vi "MyHostCode.vi"() -> ()   [LabVIEW 2017]
doc: "This VI was generated automatically using the FPGA Wizard. You can modify the VI normally."
uses:
  <vilib>/rvi/interface/nirviMethod/nirviMethod.xnode
  <vilib>/rvi/interface/nirviCloseFPGA/nirviCloseFPGA.xnode
  <vilib>/rvi/interface/nirviOpenFPGA/nirviOpenFPGA.xnode
  <vilib>/rvi/interface/nirviReadWriteControl/nirviReadWriteControl.xnode
  <vilib>/rvi/errors/niLvFpgaAdjustHostInterfaceError.vi
  <vilib>/rvi/interface/Simulation/niFpgaSimulationCallBeginRW.vi
  <vilib>/FPGAPlugInAG/Dynamic/niLvFpga_ReadFifo_Dynamic.vi
  <vilib>/rvi/errors/niLvFpgaMergeErrorWithErrorCode.vi
  HostCode.lvlib
  <vilib>/Utility/file.llb/Write To Spreadsheet File (I64).vi
  SerialComm/SerialComm.lvclass
  C:/Program Files (x86)/National Instruments/LabVIEW 2017/examples/Instrument IO/Serial/support/Serial - Settings.ctl
  FPGA Bitfiles/ECGPWMAdaptiveFi_FPGATarget2_ECGAFSPIInput_RcPp5Qijrrw.lvbitx
  FPGACode/ECG AF SPI Input.vi
  <vilib>/FPGAPlugInAG/Dynamic/niLvFpga_Reset_Dynamic.vi
  <vilib>/FPGAPlugInAG/Dynamic/niLvFpga_Run_Dynamic.vi
  <vilib>/FPGAPlugInAG/Dynamic/niLvFpga_Close_Dynamic.vi
  FPGACode/Lead Enum.ctl
  Trigger Params.ctl
  FPGACode/Channel Enum.ctl
panel:
  in  "Offset":cluster{"X":i16, "Y":i16, "Z":i16}
  in  "Beta IBP":fxp<+/-,32,-16>
  out "Pressure Data":T1(array[cluster])
  in  "ECG Gain":u16(ring)=1 items=["1"=1, "2"=2, "3"=3, "4"=4, "6"=0, "8"=5, "12"=6]
  in  "Channel":i32
  in  "Sensis\nECG Scaling":i16=1 min=1 max=100 step=1
  out "RA":i16[](graph)
  out "Trigger":i16[][](graph)
  in  "Trigger":T2={"Channel"=enum."II", "Threshold"=1000, "d/dt"=FALSE, "Invert"=FALSE}
  in  "High Pass":bool
  out "Loop Time":u32
  in  "Reset":bool
  out "Taps":dbl[](graph)
  out "Weights":dbl[](graph)
  out "WeightSum":fxp<+/-,33,19> format="%.20g"
  out "BetaProduct":fxp<+/-,32,-1> format="%.33g"
  in  "Filter Size":i16=100
  out "Invasive Blood Pressure":i16[][](graph)
  in  "Plot Info":T5={"Element"={"Lead"=enum."RA", "Filter"=FALSE}, "Element 2"={"Lead"=enum."RA", "Filter"=TRUE}, "Element 3"={"Lead"=enum."LA", "Filter"=FALSE}, "Element 4"={"Lead"=enum."LA", "Filter"=TRUE}, "Element 5"={"Lead"=enum."LL", "Filter"=FALSE}, "Element 6"={"Lead"=enum."LL", "Filter"=TRUE}, "Element 7"={"Lead"=enum."II", "Filter"=TRUE}, "Element 8"={"Lead"=enum."III", "Filter"=TRUE}}
  in  "file path (dialog if empty)":path
  in  "Record":bool
  out "Gradients":i16[][](graph)
  in  "Filter On":bool=TRUE
  out "ECG":i16[][](graph)
  out "Actual Loop Rate (Ticks)":u32
  in  "Beta":fxp<+/-,32,-16>=1.000088900582341e-11
  out "Late? Latched":bool
  in  "Start 0":bool
  in  "Loop Rate (Hz)":dbl=10000.0
  out "Calculated Rate (Hz)":dbl
  out "error out":errorcluster
  in  "Global Stop":bool
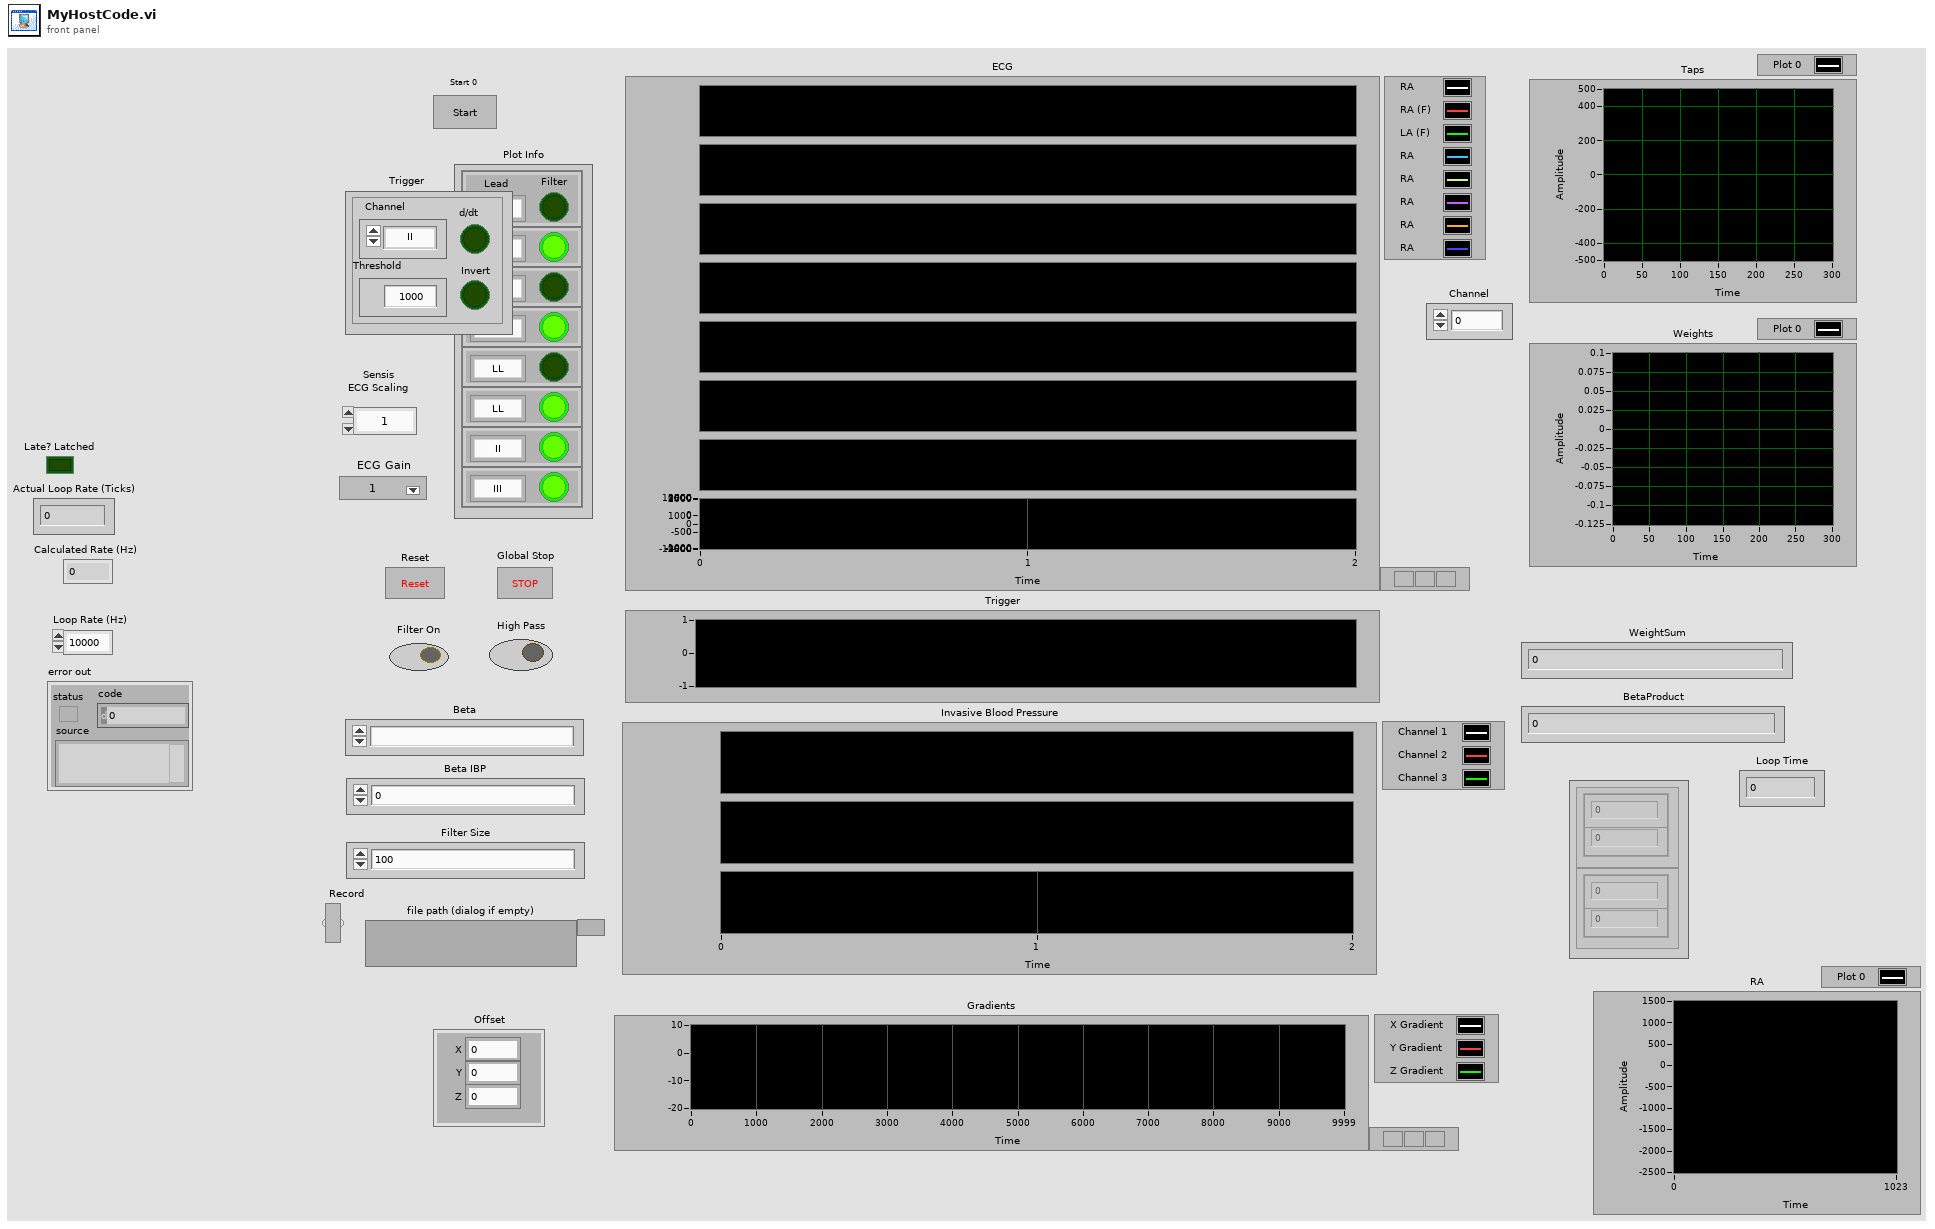
[diagram p1: front panel]
types:
  T1 = cluster{"Numeric Control":dbl, "Numeric Control":dbl}[]
  T2 = typedef "Trigger Params.ctl" = cluster{"Channel":T3, "Threshold":i16, "d/dt":bool, "Invert":bool}
  T3 = typedef "Channel Enum.ctl" = enum16{"RA", "LA", "LL", "V1", "V2", "V3", "V4", "V5", "V6", "I", "II", "III", "aVR", "aVL", "aVF", "Vw", "IBP1", "IBP2"}
  T4 = typedef "Lead Enum.ctl" = enum16{"RA", "LA", "LL", "V1", "V2", "V3", "V4", "V5", "V6", "I", "II", "III", "aVR", "aVL", "aVF", "Vw"}
  T5 = cluster{"Element":cluster{"Lead":T4, "Filter":bool}, "Element 2":cluster{"Lead":T4, "Filter":bool}, "Element 3":cluster{"Lead":T4, "Filter":bool}, "Element 4":cluster{"Lead":T4, "Filter":bool}, "Element 5":cluster{"Lead":T4, "Filter":bool}, "Element 6":cluster{"Lead":T4, "Filter":bool}, "Element 7":cluster{"Lead":T4, "Filter":bool}, "Element 8":cluster{"Lead":T4, "Filter":bool}}
  T6 = typedef "Serial - Settings.ctl" = cluster{"baud rate":u32, "data bits":u16, "parity":enum16{"None", "Odd", "Even", "Mark", "Space"}, "stop bits":u16, "flow control":u16}
  T7 = typedef "LVOffsetAndMultiplierTypeDef.ctl" = cluster{"Offset":dbl, "Multiplier":dbl}
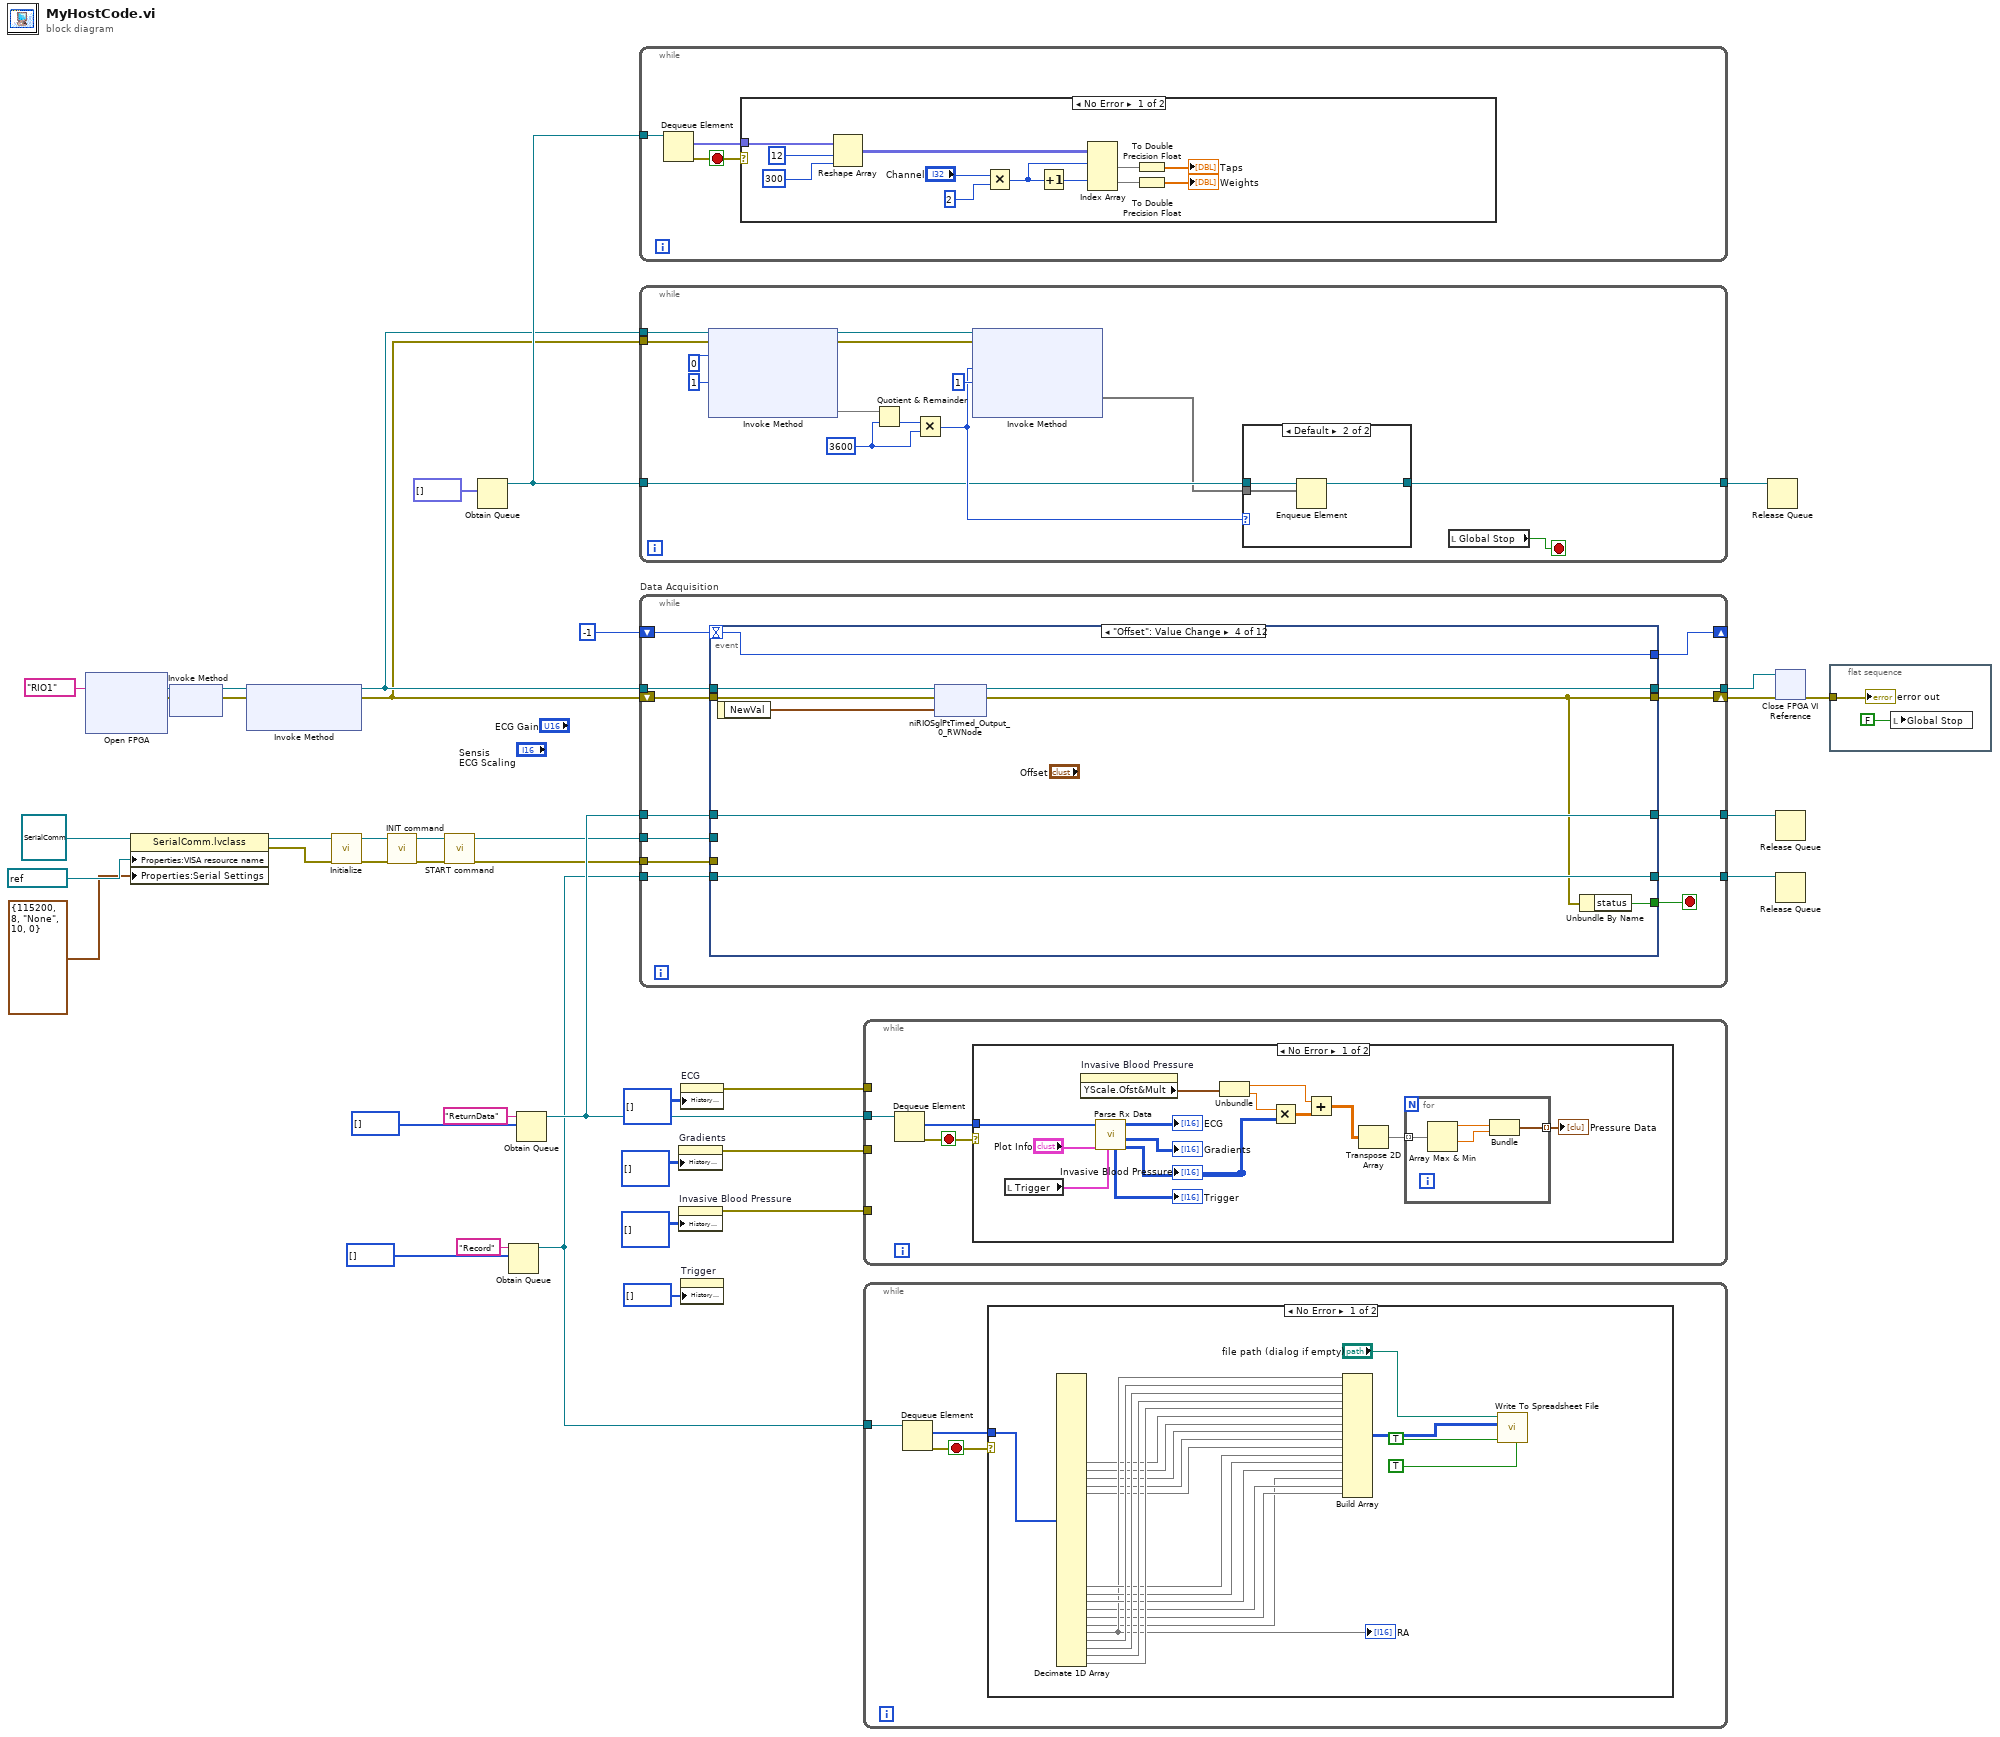
[diagram p0: block diagram]
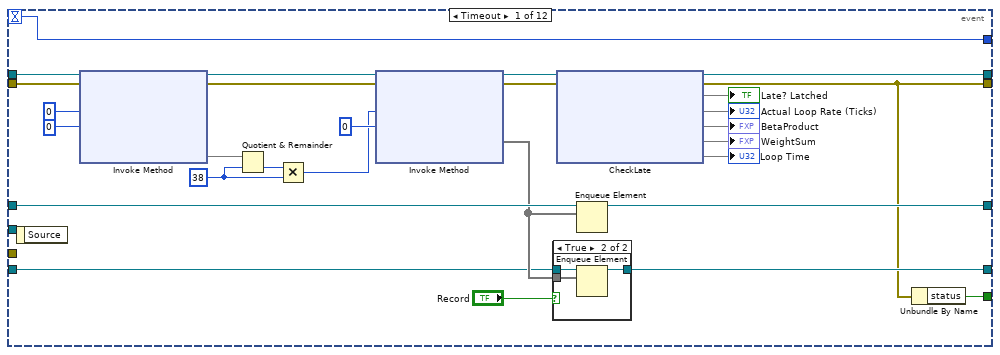
[diagram p2: hidden frame]
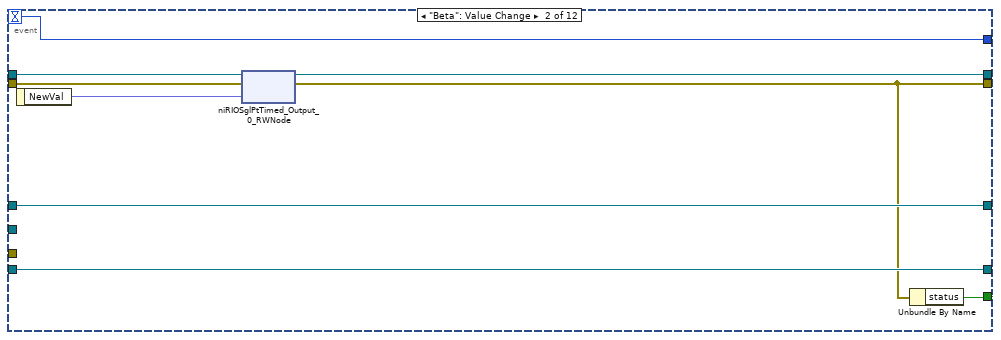
[diagram p4: hidden frame]
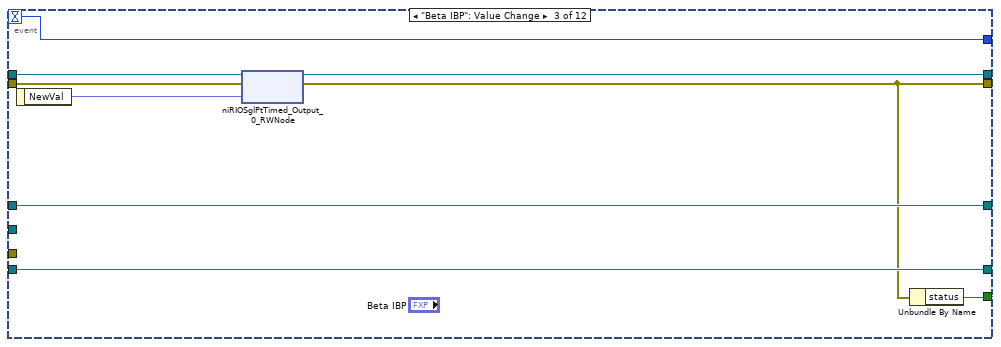
[diagram p5: hidden frame]
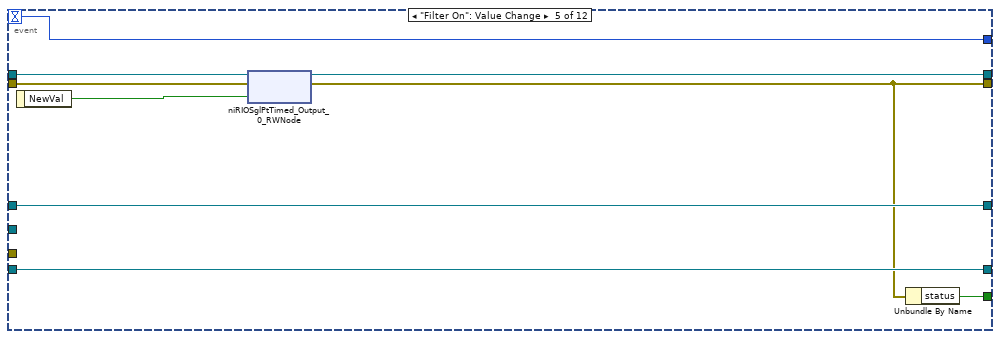
[diagram p6: hidden frame]
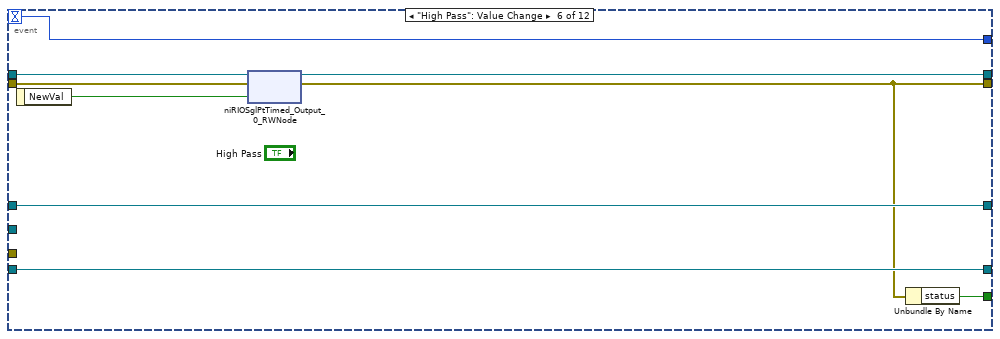
[diagram p7: hidden frame]
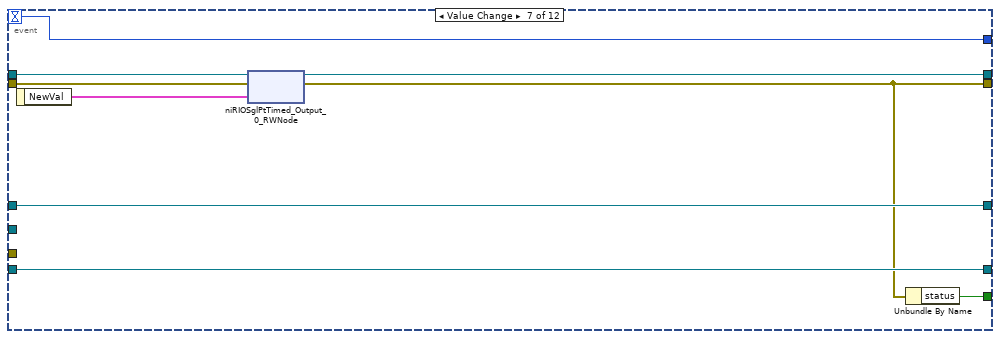
[diagram p8: hidden frame]
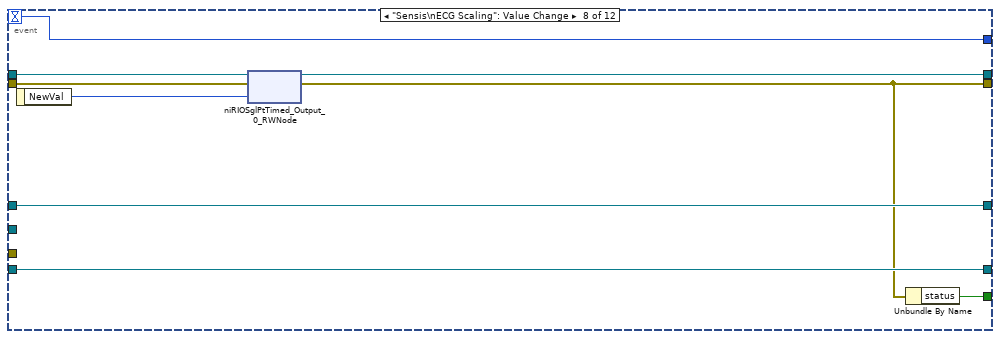
[diagram p9: hidden frame]
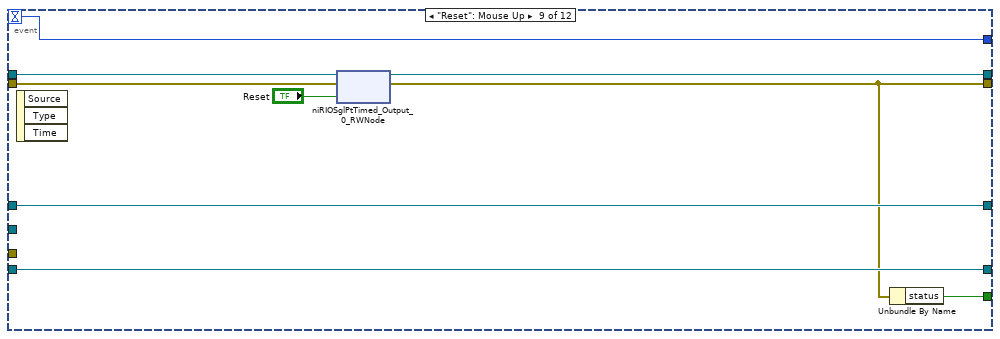
[diagram p10: hidden frame]
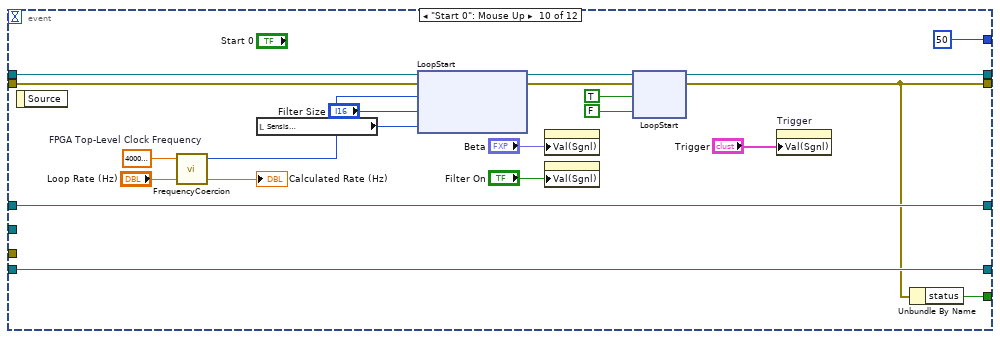
[diagram p11: hidden frame]
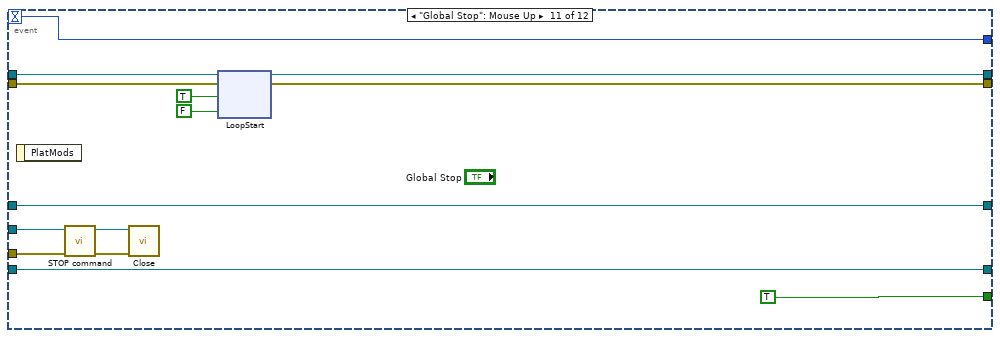
[diagram p12: hidden frame]
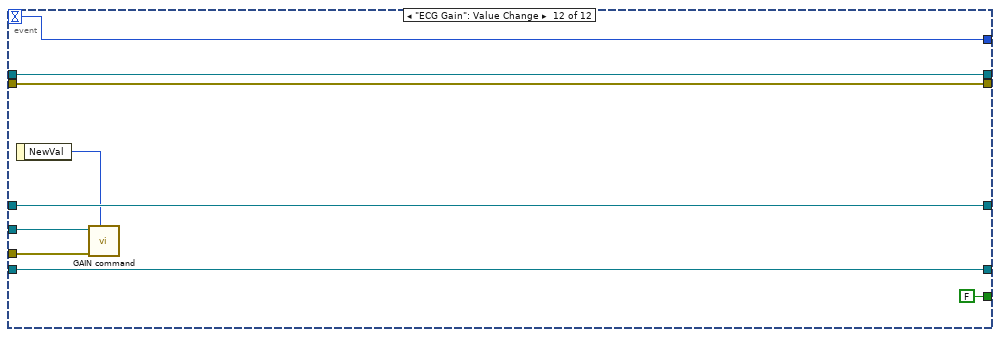
[diagram p13: hidden frame]
diagram:
  n1 = xnode ("Open FPGA")("resource name"=tag "RIO1") -> ("FPGA VI Reference Out"=w39:refnum<k20>, "error out"=w38:errorcluster)  [unwired: 1 in]
  n2 = property class="SerialComm.lvclass"(reference=refnum<class "SerialComm.lvclass"> refnum ("SerialComm.lvclass"), "Properties:VISA resource name"=refnum<visa-resource-name> "COM6" ("VISA resource name"), "Properties:Serial Settings"=T6 {"baud rate"=115200, "data bits"=8, "parity"=enum."None", "stop bits"=10, "flow control"=0} ("Serial Settings")) -> (reference out=w8:refnum<class "SerialComm.lvclass">, error out=w4:errorcluster)  [unwired: 1 in]
  n3 = xnode ("Invoke Method")("FPGA VI Reference In"=w39, "error in"=w38) -> ("FPGA VI Reference Out"=w16:refnum<k20>, "error out"=w40:errorcluster)
  n4 = xnode ("Invoke Method")("FPGA VI Reference In"=w16, "error in"=w40) -> ("FPGA VI Reference Out"=w14:refnum<k20>, "error out"=w13:errorcluster)  [unwired: 1 in]
  n5 = call "Initialize.vi"("Error In"=w4, "SerialComm in"=w8) -> ("Error Out"=w3:errorcluster, "SerialComm out"=w7:refnum<class "SerialComm.lvclass">)  [unwired: 8 in]
  n6 = call "INIT command.vi"("Error In"=w3, "SerialComm in"=w7) -> ("Error Out"=w2:errorcluster, "SerialComm out"=w6:refnum<class "SerialComm.lvclass">)  [unwired: 8 in]
  n7 = call "START command.vi"("Error In"=w2, "SerialComm in"=w6) -> ("Error Out"=w1:errorcluster, "SerialComm out"=w5:refnum<class "SerialComm.lvclass">)  [unwired: 8 in]
  n8 = Obtain Queue(element data type=fxp<+/-,32,16>[] [] ("Data")) -> (queue out=w19:refnum<queue>)  [unwired: 4 in, 2 out]
  n9 = Obtain Queue(name (unnamed)="Record", element data type=i16[] []) -> (queue out=w24:refnum<queue>)  [unwired: 3 in, 2 out]
  n10 = Obtain Queue(name (unnamed)="ReturnData", element data type=i16[] []) -> (queue out=w32:refnum<queue>)  [unwired: 3 in, 2 out]
  n11 = while {
    tunnel: w19 -> [w43]
    stop <- w41 stop-if-true
    n12 = Dequeue Element(queue=w43) -> (element=w42:fxp<+/-,32,16>[], error out=w41:errorcluster)  [unwired: 2 in, 2 out]
    n13 = case shown="No Error" w41 {
      tunnel: w42 -> [w55 _]
      frame No Error {
        n14 = Reshape Array(w55, 12 ("dimension size"), 300 ("dimension size")) -> (w51:fxp<+/-,32,16>[][])
        n15 = Multiply(x="Channel", y=2) -> (x*y=w44:i32)
        n16 = Increment(x=w44) -> (x+1=w45:i32)
        n17 = Index Array(array=w51, index (row) #1=w44, index (row) #2=w45) -> (element #1=w50:fxp<+/-,32,16>[], element #2=w49:fxp<+/-,32,16>[])  [unwired: 2 in]
        n18 = To Double Precision Float(number=w50) -> (double precision float=→"Taps":dbl[])
        n19 = To Double Precision Float(number=w49) -> (double precision float=→"Weights":dbl[])
      }
      frame Error {
      }
    }
  }
  n20 = while {
    tunnel: w14 -> [w70]
    tunnel: w13 -> [w69]
    tunnel: w19 -> [w58]
    tunnel: [w56] -> w18
    stop <- w61 stop-if-true
    w63 = u32 3600 ("y")
    n21 = xnode "Invoke Method"("FPGA VI Reference In"=w70, "error in"=w69, "Number of Elements"=u32 0, "Timeout (ms)"=1) -> ("FPGA VI Reference Out"=w66:refnum<k20>, "error out"=w65:errorcluster, "Elements Remaining"=w62)  [unwired: 1 out]
    n22 = Quotient & Remainder(x=w62, y=w63) -> (floor(x/y)=w64:u32)  [unwired: 1 out]
    n23 = Multiply(x=w64, y=w63) -> (x*y=w59:u32)
    n24 = xnode "Invoke Method"("FPGA VI Reference In"=w66, "error in"=w65, "Number of Elements"=w59, "Timeout (ms)"=1) -> ("Data"=w57:void[])  [unwired: 3 out]
    n25 = case shown="Default" w59 {
      tunnel: w58 -> [w71 w74]
      tunnel: w57 -> [_ w73]
      tunnel: [w71 w72] -> w56
      frame 0 {
      }
      frame Default {
        n26 = Enqueue Element(queue=w74, element=w73) -> (queue out=w72:refnum<queue>)  [unwired: 2 in, 2 out]
      }
    }
    n27 = local read "Global Stop"() -> (w61:bool)
  }
  n28 = while "Data Acquisition" {
    tunnel: w14 -> [w83]
    shift-right: [w87] -> w37
    shift-left: w13 -> [w84]
    tunnel: [w85] -> w35
    tunnel: w32 -> [w82]
    tunnel: [w81] -> w27
    tunnel: w24 -> [w80]
    tunnel: [w79] -> w23
    shift-right: [w77] -> _
    shift-left: -1 -> [w78]
    tunnel: w5 -> [w76]
    tunnel: w1 -> [w75]
    stop <- w86 stop-if-true
    n29 = event shown="[3] \"Offset\": Value Change" {
      selector: _ -> [_ _ _ _ _ _ _ _ _ _ _ _]
      dyn-events: _ -> [_ _ _ _ _ _ _ _ _ _ _ _]
      timeout: w78 -> [w90 w122 w131 w140 w149 w158 w167 w177 w185 _ w219 w233]
      tunnel: [w89 w121 w130 w139 w148 w157 w166 w176 w184 w195 w220 w234] -> w87
      tunnel: [w88 w120 w129 w138 w147 w156 w165 w175 w183 w194 TRUE FALSE ("status")] -> w86
      tunnel: [w115 w126 w135 w144 w153 w162 w171 w180 w189 w200 w221 w235] -> w85
      tunnel: w84 -> [w92 w127 w136 w145 w154 w163 w172 w181 w190 w210 w222 w234]
      tunnel: w83 -> [w93 w128 w137 w146 w155 w164 w173 w182 w191 w211 w223 w235]
      tunnel: w82 -> [w104 w124 w133 w142 w151 w160 w169 w179 w188 w209 w226 w232]
      tunnel: [w100 w124 w133 w142 w151 w160 w169 w179 w188 w209 w226 w232] -> w81
      tunnel: w80 -> [w97 w123 w132 w141 w150 w159 w168 w178 w187 w208 w225 w231]
      tunnel: [w91 w123 w132 w141 w150 w159 w168 w178 w187 w208 w225 w231] -> w79
      tunnel: [w90 w122 w131 w140 w149 w158 w167 w177 w185 50 w219 w233] -> w77
      tunnel: w76 -> [_ _ _ _ _ _ _ _ _ _ w216 w229]
      tunnel: w75 -> [_ _ _ _ _ _ _ _ _ _ w215 w228]
      event Timeout {
        w102 = u32 38 ("y")
        n30 = event-data() -> ()  [unwired: 1 in, 1 out]
        n31 = xnode "Invoke Method"("FPGA VI Reference In"=w93, "error in"=w92, "Number of Elements"=u32 0, "Timeout (ms)"=0) -> ("FPGA VI Reference Out"=w110:refnum<k20>, "error out"=w109:errorcluster, "Elements Remaining"=w108)  [unwired: 1 out]
        n32 = Quotient & Remainder(x=w108, y=w102) -> (floor(x/y)=w103:u32)  [unwired: 1 out]
        n33 = Multiply(x=w103, y=w102) -> (x*y=w101:u32)
        n34 = xnode "Invoke Method"("FPGA VI Reference In"=w110, "error in"=w109, "Number of Elements"=w101, "Timeout (ms)"=0) -> ("FPGA VI Reference Out"=w106:refnum<k20>, "error out"=w105:errorcluster, "Data"=w98:void[])  [unwired: 1 out]
        n35 = case shown="True" "Record" {
          tunnel: w98 -> [_ w119]
          tunnel: w97 -> [w116 w118]
          tunnel: [w116 w117] -> w91
          frame False {
          }
          frame True {
            n36 = Enqueue Element(queue=w118, element=w119) -> (queue out=w117:refnum<queue>)  [unwired: 2 in, 2 out]
          }
        }
        n37 = xnode ("CheckLate")("FPGA VI Reference In"=w106, "error in"=w105) -> ("FPGA VI Reference Out"=w115:refnum<k20>, "error out"=w89:errorcluster, "Late? Latched"=→"Late? Latched", "Actual Loop Rate (Ticks)"=→"Actual Loop Rate (Ticks)", "BetaProduct"=→"BetaProduct", "WeightSum"=→"WeightSum", "Loop Time"=→"Loop Time")
        n38 = Enqueue Element(queue=w104, element=w98) -> (queue out=w100:refnum<queue>)  [unwired: 2 in, 2 out]
        n39 = Unbundle By Name(w89) -> ("status"=w88:bool)
      }
      event "Beta": Value Change {
        n40 = event-data() -> ("NewVal"=w125:fxp<+/-,32,-16>)  [unwired: 1 in]
        n41 = xnode ("niRIOSglPtTimed_Output_0_RWNode")("FPGA VI Reference In"=w128, "error in"=w127, "Beta"=w125) -> ("FPGA VI Reference Out"=w126:refnum<k20>, "error out"=w121:errorcluster)
        n42 = Unbundle By Name(w121) -> ("status"=w120:bool)
      }
      event "Beta IBP": Value Change {
        n43 = event-data() -> ("NewVal"=w134:fxp<+/-,32,-16>)  [unwired: 1 in]
        n44 = xnode ("niRIOSglPtTimed_Output_0_RWNode")("FPGA VI Reference In"=w137, "error in"=w136, "Beta IBP"=w134) -> ("FPGA VI Reference Out"=w135:refnum<k20>, "error out"=w130:errorcluster)
        n45 = Unbundle By Name(w130) -> ("status"=w129:bool)
      }
      event "Offset": Value Change {
        n46 = event-data() -> ("NewVal"=w143:cluster{"X":i16, "Y":i16, "Z":i16})  [unwired: 1 in]
        n47 = xnode ("niRIOSglPtTimed_Output_0_RWNode")("FPGA VI Reference In"=w146, "error in"=w145, "Offset"=w143) -> ("FPGA VI Reference Out"=w144:refnum<k20>, "error out"=w139:errorcluster)
        n48 = Unbundle By Name(w139) -> ("status"=w138:bool)
      }
      event "Filter On": Value Change {
        n49 = event-data() -> ("NewVal"=w152:bool)  [unwired: 1 in]
        n50 = xnode ("niRIOSglPtTimed_Output_0_RWNode")("FPGA VI Reference In"=w155, "error in"=w154, "Filter On"=w152) -> ("FPGA VI Reference Out"=w153:refnum<k20>, "error out"=w148:errorcluster)
        n51 = Unbundle By Name(w148) -> ("status"=w147:bool)
      }
      event "High Pass": Value Change {
        n52 = event-data() -> ("NewVal"=w161:bool)  [unwired: 1 in]
        n53 = xnode ("niRIOSglPtTimed_Output_0_RWNode")("FPGA VI Reference In"=w164, "error in"=w163, "HPF"=w161) -> ("FPGA VI Reference Out"=w162:refnum<k20>, "error out"=w157:errorcluster)
        n54 = Unbundle By Name(w157) -> ("status"=w156:bool)
      }
      event Value Change {
        n55 = event-data() -> ("NewVal"=w170:T2)  [unwired: 1 in]
        n56 = xnode ("niRIOSglPtTimed_Output_0_RWNode")("FPGA VI Reference In"=w173, "error in"=w172, "Trigger"=w170) -> ("FPGA VI Reference Out"=w171:refnum<k20>, "error out"=w166:errorcluster)
        n57 = Unbundle By Name(w166) -> ("status"=w165:bool)
      }
      event "Sensis\nECG Scaling": Value Change {
        n58 = event-data() -> ("NewVal"=w174:i16)  [unwired: 1 in]
        n59 = xnode ("niRIOSglPtTimed_Output_0_RWNode")("FPGA VI Reference In"=w182, "error in"=w181, "Scale"=w174) -> ("FPGA VI Reference Out"=w180:refnum<k20>, "error out"=w176:errorcluster)
        n60 = Unbundle By Name(w176) -> ("status"=w175:bool)
      }
      event "Reset": Mouse Up {
        n61 = event-data() -> ()  [unwired: 1 in, 3 out]
        n62 = xnode ("niRIOSglPtTimed_Output_0_RWNode")("FPGA VI Reference In"=w191, "error in"=w190, "Reset"="Reset") -> ("FPGA VI Reference Out"=w189:refnum<k20>, "error out"=w184:errorcluster)
        n63 = Unbundle By Name(w184) -> ("status"=w183:bool)
      }
      event "Start 0": Mouse Up {
        w207 = 40000000.0  # FPGA Top-Level Clock Frequency
        n64 = event-data() -> ()  [unwired: 1 in, 1 out]
        n65 = call "FrequencyCoercion.vi"("Loop Rate (Hz)"="Loop Rate (Hz)", "FPGA Top-Level Clock Frequency"=w207) -> ("Actual Rate (Hz)"=→"Calculated Rate (Hz)":dbl, "FPGA Ticks"=w204:u32)  [unwired: 2 in]
        n66 = local read "Sensis\nECG Scaling"() -> (w192:i16)
        n67 = xnode ("LoopStart")("FPGA VI Reference In"=w211, "error in"=w210, "Loop Rate (Ticks)"=w204, "Filter Size"="Filter Size", "Scale"=w192) -> ("FPGA VI Reference Out"=w202:refnum<k20>, "error out"=w201:errorcluster)
        n68 = property on="Beta" class="DigNum (strict)"("Val(Sgnl)"="Beta") -> ()  [unwired: 2 in, 2 out]
        n69 = property on="Filter On" class="Bool (strict)"("Val(Sgnl)"="Filter On") -> ()  [unwired: 2 in, 2 out]
        n70 = xnode ("LoopStart")("FPGA VI Reference In"=w202, "error in"=w201, "Start 0"=TRUE, "Start 0"=FALSE) -> ("FPGA VI Reference Out"=w200:refnum<k20>, "error out"=w195:errorcluster)
        n71 = property on="Trigger" class="Clust (strict)"("Val(Sgnl)"="Trigger") -> ()  [unwired: 2 in, 2 out]
        n72 = Unbundle By Name(w195) -> ("status"=w194:bool)
      }
      event "Global Stop": Mouse Up {
        n73 = event-data() -> ()  [unwired: 1 in, 1 out]
        n74 = call "STOP command.vi"("Error In"=w215, "SerialComm in"=w216) -> ("Error Out"=w213:errorcluster, "SerialComm out"=w214:refnum<class "SerialComm.lvclass">)  [unwired: 8 in]
        n75 = call "Close.vi"("Error In"=w213, "SerialComm in"=w214) -> ()  [unwired: 8 in, 2 out]
        n76 = xnode ("LoopStart")("FPGA VI Reference In"=w223, "error in"=w222, "stop"=TRUE, "stop"=FALSE) -> ("FPGA VI Reference Out"=w221:refnum<k20>, "error out"=w220:errorcluster)
      }
      event "ECG Gain": Value Change {
        n77 = event-data() -> ("NewVal"=w227:u16)  [unwired: 1 in]
        n78 = call "GAIN command.vi"("Ring"=w227, "Error In"=w228, "SerialComm in"=w229) -> ()  [unwired: 7 in, 2 out]
      }
    }
  }
  n79 = property on="Gradients" class="WFChart (strict)"("History Data"=i16[][] []) -> (error out=w29:errorcluster)  [unwired: 2 in, 1 out]
  n80 = property on="Invasive Blood Pressure" class="WFChart (strict)"("History Data"=i16[][] []) -> (error out=w21:errorcluster)  [unwired: 2 in, 1 out]
  n81 = property on="ECG" class="WFChart (strict)"("History Data"=i16[][] []) -> (error out=w30:errorcluster)  [unwired: 2 in, 1 out]
  n82 = property on="Trigger" class="WFChart (strict)"("History Data"=i16[] []) -> ()  [unwired: 2 in, 2 out]
  n83 = while {
    tunnel: w32 -> [w238]
    tunnel: w30 -> [_]
    tunnel: w29 -> [_]
    tunnel: w21 -> [_]
    stop <- w237 stop-if-true
    n84 = Dequeue Element(queue=w238) -> (element=w236:i16[], error out=w237:errorcluster)  [unwired: 2 in, 2 out]
    n85 = case shown="No Error" w237 {
      tunnel: w236 -> [w252 _]
      frame No Error {
        n86 = local read "Trigger"() -> (w249:T2)
        n87 = property on="Invasive Blood Pressure" class="WFChart (strict)"() -> ("YScale.Ofst&Mult"=w244:T7)  [unwired: 2 in, 2 out]
        n88 = call "Parse Rx Data.vi"("Trigger"=w249, "Plot Info"="Plot Info", "Input Data"=w252) -> ("Pressures"=w243:i16[][], "Gradients"=→"Gradients":i16[][], "ECG Data"=→"ECG":i16[][], "Trigger"=→"Trigger":i16[][])  [unwired: 5 in]
        "Invasive Blood Pressure" <- w243
        n89 = Unbundle(w244) -> ("Offset"=w240:dbl, "Multiplier"=w242:dbl)
        n90 = Multiply(x=w242, y=w243) -> (x*y=w241:dbl[][])
        n91 = Add(x=w240, y=w241) -> (x+y=w239:dbl[][])
        n92 = Transpose 2D Array(2D array=w239) -> (transposed array=w245:dbl[][])
        n93 = for {
          tunnel: w245 -> [w256] mode=indexing
          tunnel: [w253] -> w246 mode=indexing
          n94 = Array Max & Min(array=w256) -> (max value=w255:dbl, min value=w254:dbl)  [unwired: 2 out]
          n95 = Bundle(w255, w254) -> (w253:cluster{dbl, dbl})  [unwired: 1 in]
        }
        "Pressure Data" <- w246
      }
      frame Error {
      }
    }
  }
  n96 = while {
    tunnel: w24 -> [w257]
    stop <- w259 stop-if-true
    n97 = Dequeue Element(queue=w257) -> (element=w258:i16[], error out=w259:errorcluster)  [unwired: 2 in, 2 out]
    n98 = case shown="No Error" w259 {
      tunnel: w258 -> [w277 _]
      frame No Error {
        n99 = Decimate 1D Array(w277) -> (w267:i16[], w266:i16[], w265:i16[], w264:i16[], w263:i16[], w270:i16[], w271:i16[], w272:i16[], w261:i16[], w262:i16[], w260:i16[], w268:i16[], w276:i16[], w275:i16[], w274:i16[], w273:i16[])  [unwired: 22 out]
        "RA" <- w268
        n100 = Build Array(w268, w276, w275, w274, w273, w267, w266, w265, w264, w263, w270, w271, w272, w260, w261, w262) -> (w269:i16[][])
        n101 = call-poly <vilib>:"Write To Spreadsheet File.vi"("transpose? (no:F)"=TRUE, "append to file? (new file:F)"=TRUE, "2D data"=w269, "file path (dialog if empty)"="file path (dialog if empty)") -> ()  [unwired: 4 in, 1 out]
      }
      frame Error {
      }
    }
  }
  n102 = Release Queue(queue=w18) -> ()  [unwired: 2 in, 3 out]
  n103 = xnode ("Close FPGA VI Reference")("FPGA VI Reference In"=w35, "error in"=w37) -> ("error out"=w36:errorcluster)
  n104 = Release Queue(queue=w27) -> ()  [unwired: 2 in, 3 out]
  n105 = Release Queue(queue=w23) -> ()  [unwired: 2 in, 3 out]
  n106 = flat-sequence {
    tunnel: w36 -> [w282]
    frame #0 {
      n107 = local write "Global Stop"(FALSE ("Global Stop")) -> ()
      "error out" <- w282
    }
  }
